vi "Point Data Updated.vi"(8 "error in":errorcluster, 9 "Data":variant, 10 "Point Ident":string, 11 "Sample PWM Fans in":refnum<class "Sample PWM Fans.lvclass">) -> (0 "error out":errorcluster, 3 "Sample PWM Fans out":refnum<class "Sample PWM Fans.lvclass">)   [LabVIEW 2023, in "Sample PWM Fans.lvlib" / "Sample PWM Fans.lvclass"]
doc: "Use this VI to update Point Data for repeatedly self calling Do.VI's"
uses:
  Sample PWM Fans.lvclass
  Sample PWM Fans.lvclass/Sample PWM Fans.ctl
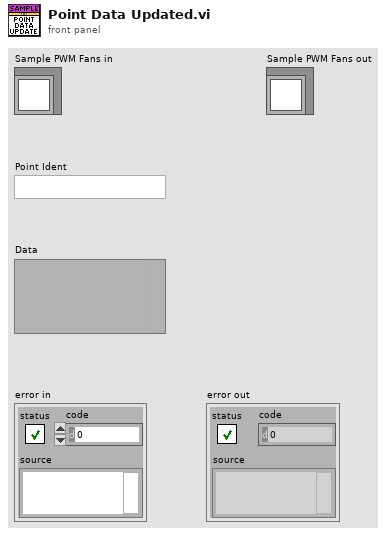
[diagram p1: front panel]
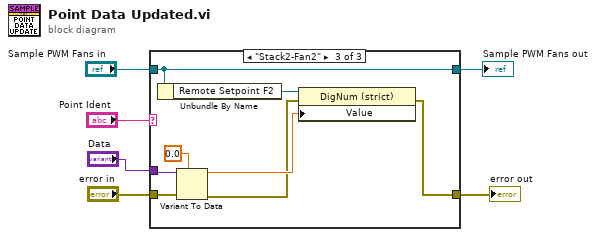
[diagram p0: block diagram]
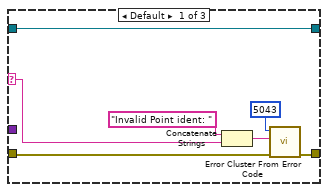
[diagram p2: hidden frame]
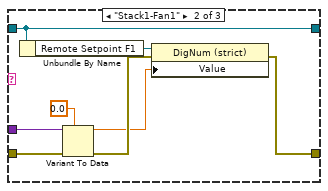
[diagram p3: hidden frame]
diagram:
  n1 = case shown="\"Stack2-Fan2\"" "Point Ident" {
    selector: "Point Ident" -> [w8 _ _]
    tunnel: "Sample PWM Fans in" -> [w13 w21 w29]
    tunnel: [w13 w21 w29] -> w4
    tunnel: [w12 w19 w22] -> w3
    tunnel: "error in" -> [w11 w18 w27]
    tunnel: "Data" -> [_ w16 w26]
    frame Default {
      n2 = Concatenate Strings("Invalid Point ident: " ("string"), w8) -> (w7:string)
      n3 = call <vilib>:"Error Cluster From Error Code.vi"("error in (no error)"=w11, "error message (\"\")"=w7, "error code (0)"=5043) -> ("error out"=w12:errorcluster)  [unwired: 6 in]
    }
    frame "Stack1-Fan1" {
      n4 = Unbundle By Name(w21) -> ("Remote Setpoint F1"=w20:refnum<vi>)
      n5 = Variant To Data(error in=w18, type=0.0, Variant=w16) -> (data=w14:dbl, error out=w17:errorcluster)
      n6 = property class="DigNum (strict)"(reference=w20, error in=w17, "Value"=w14) -> (error out=w19:errorcluster)  [unwired: 1 out]
    }
    frame "Stack2-Fan2" {
      n7 = Unbundle By Name(w29) -> ("Remote Setpoint F2"=w28:refnum<vi>)
      n8 = Variant To Data(error in=w27, type=0.0, Variant=w26) -> (data=w24:dbl, error out=w23:errorcluster)
      n9 = property class="DigNum (strict)"(reference=w28, error in=w23, "Value"=w24) -> (error out=w22:errorcluster)  [unwired: 1 out]
    }
  }
  "error out" <- w3
  "Sample PWM Fans out" <- w4
